vi "SendQueueMessage_Cluster.vi"(6 "timeout in ms (-1)":i32=-1, 8 "error in":errorcluster, 10 "message":T1, 11 "message ref in":refnum<class "CLM_LocalMessage_Queue.lvclass">) -> (0 "error out":errorcluster, 3 "message ref out":refnum<class "CLM_LocalMessage_Queue.lvclass">, 4 "timed out?":bool)   [LabVIEW 2013, in "CLM_LocalMessage_Queue.lvclass"]
uses:
  CLM_LocalMessage_Queue.lvclass
  LocalMessage/Message.ctl
  CLM_LocalMessage_Queue.lvclass/CLM_LocalMessage_Queue.ctl
  LocalMessage/CLM_LocalMessage.lvclass
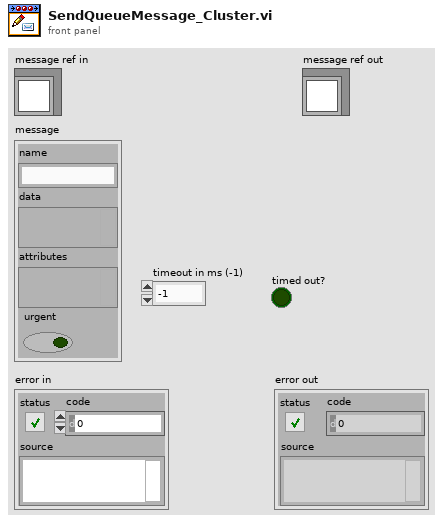
[diagram p1: front panel]
types:
  T1 = typedef "CLM_LocalMessage.lvclass/Message.ctl" = cluster{"name":string, "data":variant, "attributes":variant, "urgent":bool}
  T2 = typedef "CLM_LocalMessage_Queue.lvclass/MessageQueue.ctl" = refnum<queue>
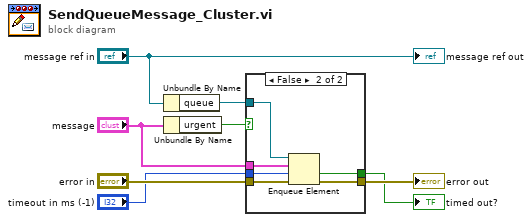
[diagram p0: block diagram]
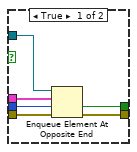
[diagram p2: hidden frame]
diagram:
  n1 = Unbundle By Name("message ref in") -> ("queue"=w1:T2)
  n2 = Unbundle By Name("message") -> ("urgent"=w8:bool)
  n3 = case shown="False" w8 {
    tunnel: "error in" -> [w14 w20]
    tunnel: w1 -> [w13 w19]
    tunnel: "message" -> [w12 w18]
    tunnel: [w11 w17] -> w5
    tunnel: "timeout in ms (-1)" -> [w10 w16]
    tunnel: [w9 w15] -> w3
    frame True {
      n4 = Enqueue Element At Opposite End(queue=w13, element=w12, timeout in ms (-1)=w10, error in (no error)=w14) -> (timed out?=w9:bool, error out=w11:errorcluster)  [unwired: 1 out]
    }
    frame False {
      n5 = Enqueue Element(queue=w19, element=w18, timeout in ms (-1)=w16, error in (no error)=w20) -> (timed out?=w15:bool, error out=w17:errorcluster)  [unwired: 1 out]
    }
  }
  "error out" <- w5
  "timed out?" <- w3
  "message ref out" <- "message ref in"
